vi "17_2.vi"() -> ()   [LabVIEW 2018]
panel:
  out "x-y":u32
  out "sum":i16=2552
  out "Array 2":bool[][][][](array[boolean])
  in  "Input":string="##...#.#\n####.#.#\n#...####\n..#.#.#.\n####.#..\n#.#.#..#\n.####.##\n..#...##"
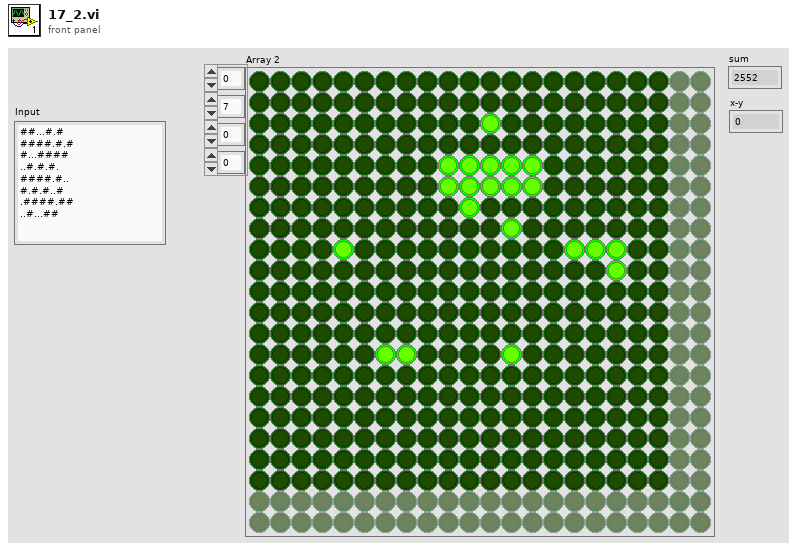
[diagram p1: front panel]
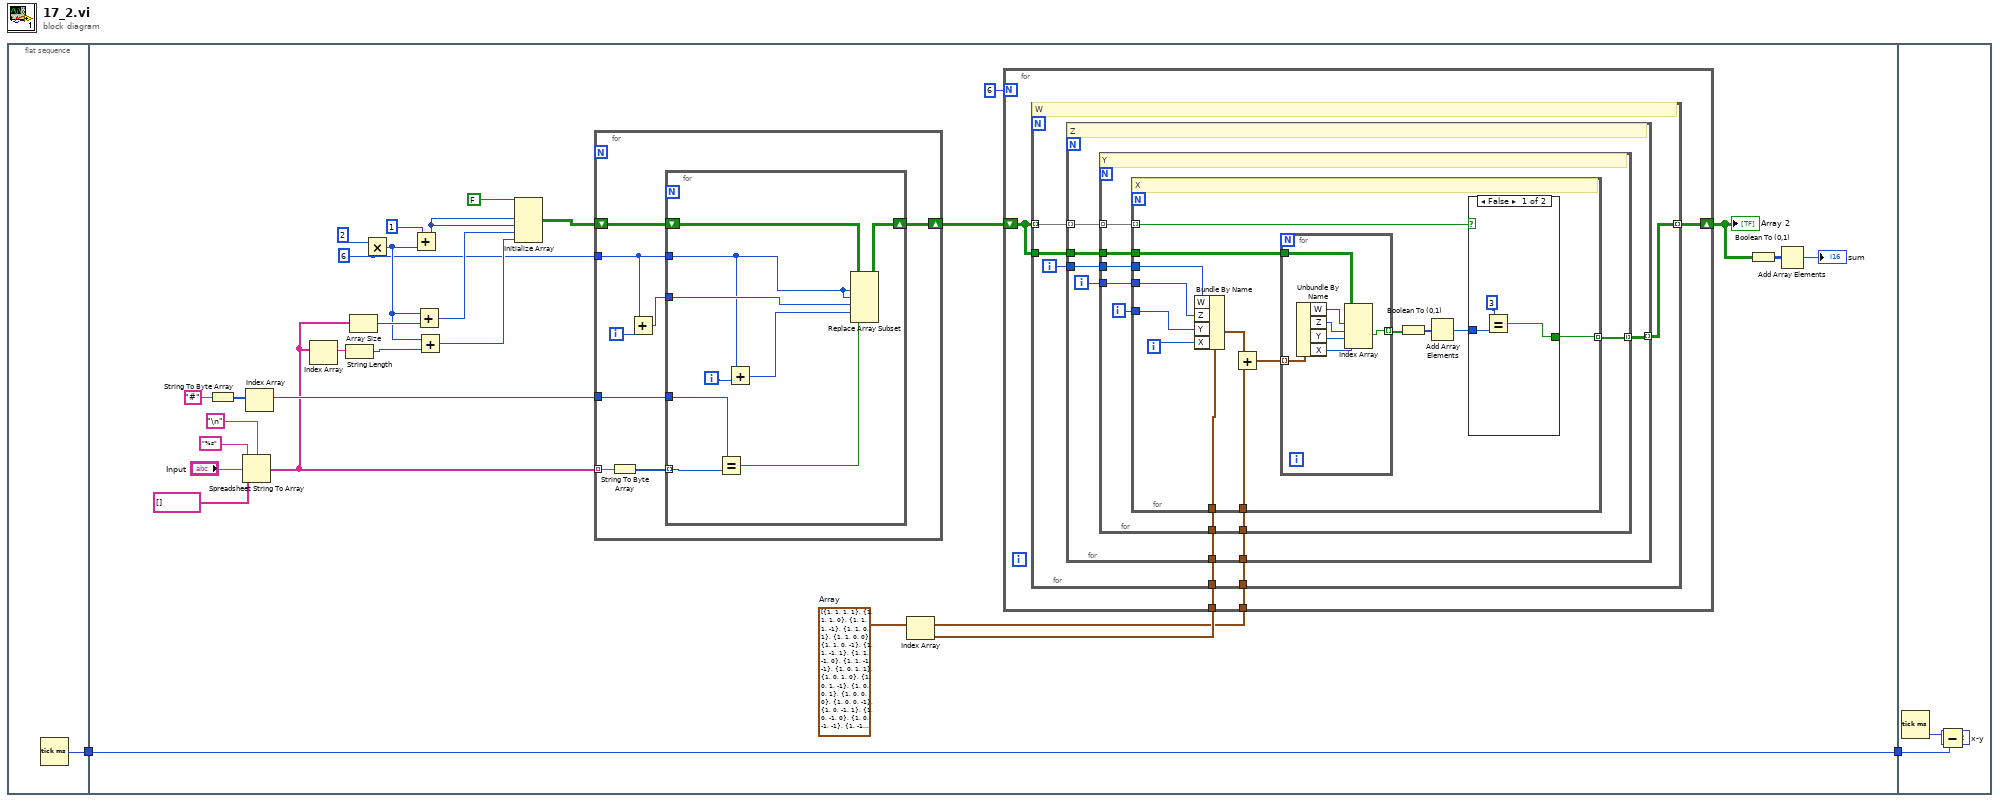
[diagram p0: block diagram]
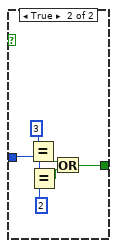
[diagram p2: hidden frame]
diagram:
  n1 = flat-sequence {
    tunnel: [w3] -> w2
    tunnel: w2 -> [w4]
    tunnel: [w4] -> w1
    tunnel: w1 -> [w105]
    frame #0 {
      n2 = Tick Count (ms)() -> (millisecond timer value=w3:u32)
    }
    frame #1 {
      w5 = cluster{"W":i32, "Z":i32, "Y":i32, "X":i32}[] [{"W"=1, "Z"=1, "Y"=1, "X"=1}, {"W"=1, "Z"=1, "Y"=1, "X"=0}, {"W"=1, "Z"=1, "Y"=1, "X"=-1}, {"W"=1, "Z"=1, "Y"=0, "X"=1}, {"W"=1, "Z"=1, "Y"=0, "X"=0}, {"W"=1, "Z"=1, "Y"=0, "X"=-1}, {"W"=1, "Z"=1, "Y"=-1, "X"=1}, {"W"=1, "Z"=1, "Y"=-1, "X"=0}, {"W"=1, "Z"=1, "Y"=-1, "X"=-1}, {"W"=1, "Z"=0, "Y"=1, "X"=1}, {"W"=1, "Z"=0, "Y"=1, "X"=0}, {"W"=1, "Z"=0, "Y"=1, "X"=-1}, {"W"=1, "Z"=0, "Y"=0, "X"=1}, {"W"=1, "Z"=0, "Y"=0, "X"=0}, {"W"=1, "Z"=0, "Y"=0, "X"=-1}, {"W"=1, "Z"=0, "Y"=-1, "X"=1}, {"W"=1, "Z"=0, "Y"=-1, "X"=0}, {"W"=1, "Z"=0, "Y"=-1, "X"=-1}, {"W"=1, "Z"=-1, "Y"=1, "X"=1}, {"W"=1, "Z"=-1, "Y"=1, "X"=0}, {"W"=1, "Z"=-1, "Y"=1, "X"=-1}, {"W"=1, "Z"=-1, "Y"=0, "X"=1}, {"W"=1, "Z"=-1, "Y"=0, "X"=0}, {"W"=1, "Z"=-1, "Y"=0, "X"=-1}, {"W"=1, "Z"=-1, "Y"=-1, "X"=1}, {"W"=1, "Z"=-1, "Y"=-1, "X"=0}, {"W"=1, "Z"=-1, "Y"=-1, "X"=-1}, {"W"=0, "Z"=1, "Y"=1, "X"=1}, {"W"=0, "Z"=1, "Y"=1, "X"=0}, {"W"=0, "Z"=1, "Y"=1, "X"=-1}, {"W"=0, "Z"=1, "Y"=0, "X"=1}, {"W"=0, "Z"=1, "Y"=0, "X"=0}, {"W"=0, "Z"=1, "Y"=0, "X"=-1}, {"W"=0, "Z"=1, "Y"=-1, "X"=1}, {"W"=0, "Z"=1, "Y"=-1, "X"=0}, {"W"=0, "Z"=1, "Y"=-1, "X"=-1}, {"W"=0, "Z"=0, "Y"=1, "X"=1}, {"W"=0, "Z"=0, "Y"=1, "X"=0}, {"W"=0, "Z"=0, "Y"=1, "X"=-1}, {"W"=0, "Z"=0, "Y"=0, "X"=1}, {"W"=0, "Z"=0, "Y"=0, "X"=-1}, {"W"=0, "Z"=0, "Y"=-1, "X"=1}, {"W"=0, "Z"=0, "Y"=-1, "X"=0}, {"W"=0, "Z"=0, "Y"=-1, "X"=-1}, {"W"=0, "Z"=-1, "Y"=1, "X"=1}, {"W"=0, "Z"=-1, "Y"=1, "X"=0}, {"W"=0, "Z"=-1, "Y"=1, "X"=-1}, {"W"=0, "Z"=-1, "Y"=0, "X"=1}, {"W"=0, "Z"=-1, "Y"=0, "X"=0}, {"W"=0, "Z"=-1, "Y"=0, "X"=-1}, {"W"=0, "Z"=-1, "Y"=-1, "X"=1}, {"W"=0, "Z"=-1, "Y"=-1, "X"=0}, {"W"=0, "Z"=-1, "Y"=-1, "X"=-1}, {"W"=-1, "Z"=1, "Y"=1, "X"=1}, {"W"=-1, "Z"=1, "Y"=1, "X"=0}, {"W"=-1, "Z"=1, "Y"=1, "X"=-1}, {"W"=-1, "Z"=1, "Y"=0, "X"=1}, {"W"=-1, "Z"=1, "Y"=0, "X"=0}, {"W"=-1, "Z"=1, "Y"=0, "X"=-1}, {"W"=-1, "Z"=1, "Y"=-1, "X"=1}, {"W"=-1, "Z"=1, "Y"=-1, "X"=0}, {"W"=-1, "Z"=1, "Y"=-1, "X"=-1}, {"W"=-1, "Z"=0, "Y"=1, "X"=1}, {"W"=-1, "Z"=0, "Y"=1, "X"=0}, {"W"=-1, "Z"=0, "Y"=1, "X"=-1}, {"W"=-1, "Z"=0, "Y"=0, "X"=1}, {"W"=-1, "Z"=0, "Y"=0, "X"=0}, {"W"=-1, "Z"=0, "Y"=0, "X"=-1}, {"W"=-1, "Z"=0, "Y"=-1, "X"=1}, {"W"=-1, "Z"=0, "Y"=-1, "X"=0}, {"W"=-1, "Z"=0, "Y"=-1, "X"=-1}, {"W"=-1, "Z"=-1, "Y"=1, "X"=1}, {"W"=-1, "Z"=-1, "Y"=1, "X"=0}, {"W"=-1, "Z"=-1, "Y"=1, "X"=-1}, {"W"=-1, "Z"=-1, "Y"=0, "X"=1}, {"W"=-1, "Z"=-1, "Y"=0, "X"=0}, {"W"=-1, "Z"=-1, "Y"=0, "X"=-1}, {"W"=-1, "Z"=-1, "Y"=-1, "X"=1}, {"W"=-1, "Z"=-1, "Y"=-1, "X"=0}, {"W"=-1, "Z"=-1, "Y"=-1, "X"=-1}]  # Array
      w13 = 6
      n3 = String To Byte Array(string="#") -> (unsigned byte array=w26:u8[])
      n4 = Spreadsheet String To Array(delimiter (Tab)="\n", format string="%s", spreadsheet string="Input", array type (2D Dbl)=string[] []) -> (array=w19:string[])
      n5 = Index Array(array=w26) -> (element=w25:u8)  [unwired: 1 in]
      n6 = Index Array(array=w19) -> (element=w18:string)  [unwired: 1 in]
      n7 = String Length(string=w18) -> (length=w17:i32)
      n8 = Array Size(array=w19) -> (size(s)=w23:i32)
      n9 = Multiply(x=2, y=w13) -> (x*y=w16:i32)
      n10 = Add(x=1, y=w16) -> (x+y=w6:i32)
      n11 = Add(x=w16, y=w23) -> (x+y=w20:i32)
      n12 = Add(x=w16, y=w17) -> (x+y=w15:i32)
      n13 = Initialize Array(FALSE, w6, w6, w20, w15) -> (w14:bool[][][][])
      n14 = for {
        tunnel: w19 -> [w94] mode=indexing
        tunnel: w25 -> [w92]
        shift-right: [w90] -> w12
        shift-left: w14 -> [w91]
        tunnel: w13 -> [w88]
        i -> [w89]
        n15 = String To Byte Array(string=w94) -> (unsigned byte array=w93:u8[])
        n16 = Add(x=w88, y=w89) -> (x+y=w87:i32)
        n17 = for {
          tunnel: w93 -> [w103] mode=indexing
          tunnel: w92 -> [w102]
          shift-right: [w100] -> w90
          shift-left: w91 -> [w101]
          tunnel: w88 -> [w95]
          tunnel: w87 -> [w96]
          i -> [w98]
          n18 = Equal?(x=w102, y=w103) -> (x = y?=w99:bool)
          n19 = Add(x=w95, y=w98) -> (x+y=w97:i32)
          n20 = Replace Array Subset(array=w101, new element=w99, index (dim 0)=w95, index (dim 1)=w95, index (dim 2)=w96, index (dim 3)=w97) -> (w100:bool[][][][])
        }
      }
      n21 = Index Array(array=w5) -> (element=w11:cluster{"W":i32, "Z":i32, "Y":i32, "X":i32})  [unwired: 1 in]
      n22 = for {
        N: 6 -> [_]
        tunnel: w11 -> [w35]
        tunnel: w5 -> [w34]
        shift-right: [w33] -> w8
        shift-left: w12 -> [w32]
        n23 = for {
          tunnel: w35 -> [w41]
          tunnel: w34 -> [w40]
          tunnel: [w39] -> w33 mode=indexing
          tunnel: w32 -> [w38] mode=indexing
          tunnel: w32 -> [w37]
          i -> [w36]
          # "W"
          n24 = for {
            tunnel: w38 -> [w48] mode=indexing
            tunnel: w37 -> [w47]
            tunnel: w41 -> [w46]
            tunnel: w40 -> [w44]
            tunnel: [w43] -> w39 mode=indexing
            tunnel: w36 -> [w42]
            i -> [w45]
            # "Z"
            n25 = for {
              tunnel: w48 -> [w56] mode=indexing
              tunnel: w47 -> [w55]
              tunnel: w46 -> [w54]
              tunnel: w45 -> [w52]
              tunnel: w44 -> [w51]
              tunnel: [w50] -> w43 mode=indexing
              tunnel: w42 -> [w49]
              i -> [w53]
              # "Y"
              n26 = for {
                tunnel: w56 -> [w62] mode=indexing
                tunnel: w55 -> [w63]
                tunnel: w54 -> [w70]
                tunnel: w53 -> [w68]
                tunnel: w52 -> [w67]
                tunnel: w51 -> [w65]
                tunnel: [w58] -> w50 mode=indexing
                tunnel: w49 -> [w57]
                i -> [w69]
                # "X"
                n27 = Bundle By Name(cluster=w70, "W"=w57, "Z"=w67, "Y"=w68, "X"=w69) -> (w66:cluster{"W":i32, "Z":i32, "Y":i32, "X":i32})
                n28 = Add(x=w66, y=w65) -> (x+y=w64:cluster{"W":i32, "Z":i32, "Y":i32, "X":i32}[])
                n29 = for {
                  tunnel: w64 -> [w85] mode=indexing
                  tunnel: w63 -> [w86]
                  tunnel: [w84] -> w61 mode=indexing
                  n30 = Unbundle By Name(w85) -> ("W"=w80:i32, "Z"=w81:i32, "Y"=w82:i32, "X"=w83:i32)
                  n31 = Index Array(array=w86, index (dim 0)=w80, index (dim 1)=w81, index (dim 2)=w82, index (dim 3)=w83) -> (element=w84:bool)
                }
                n32 = Boolean To (0,1)(Boolean=w61) -> (0, 1=w60:i16[])
                n33 = Add Array Elements(numeric array=w60) -> (sum=w59:i16)
                n34 = case shown="False" w62 {
                  tunnel: w59 -> [w72 w79]
                  tunnel: [w71 w74] -> w58
                  frame False {
                    n35 = Equal?(x=i16 3, y=w72) -> (x = y?=w71:bool)
                  }
                  frame True {
                    n36 = Equal?(x=i16 3, y=w79) -> (x = y?=w76:bool)
                    n37 = Equal?(x=w79, y=i16 2) -> (x = y?=w75:bool)
                    n38 = Or(x=w76, y=w75) -> (x .or. y?=w74:bool)
                  }
                }
              }
            }
          }
        }
      }
      "Array 2" <- w8
      n39 = Boolean To (0,1)(Boolean=w8) -> (0, 1=w9:i16[][][][])
      n40 = Add Array Elements(numeric array=w9) -> (sum=→"sum":i16)
    }
    frame #2 {
      n41 = Tick Count (ms)() -> (millisecond timer value=w106:u32)
      n42 = Subtract(x=w106, y=w105) -> (x-y=→"x-y":u32)
    }
  }
